vi "Untitled 8 (SubVI).vi"() -> (2 "time string":string, 3 "date string":string)   [LabVIEW 2017]
panel:
  out "index of element":i32
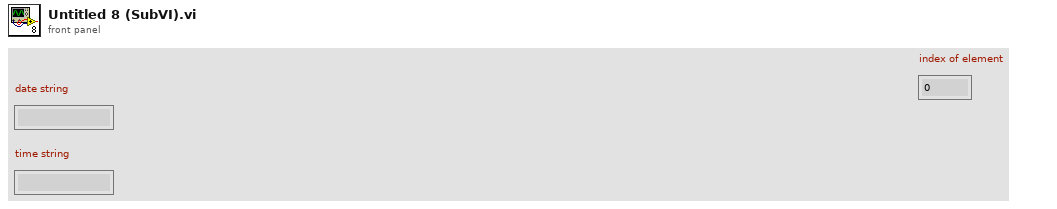
[diagram p1: front panel]
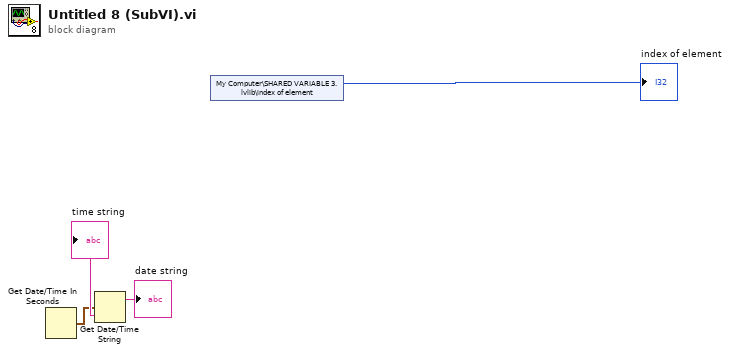
[diagram p0: block diagram]
diagram:
  n1 = Get Date/Time In Seconds() -> (seconds since 1Jan1904=w2:timestamp)
  n2 = Get Date/Time String(seconds (now)=w2) -> (date string=→"date string":string, time string=→"time string":string)  [unwired: 2 in]
  n3 = shared-variable "My Computer\\SHARED VARIABLE 3.lvlib\\index of element"() -> (→"index of element":i32)  [unwired: 1 in, 1 out]
